vi "VFH Vi.vi"(0 "LIDAR & Vision magn. (m)":dbl[](array[numeric]), 5 "LIDAR & Vision angle (rad)":dbl[](array[numeric]), 7 "current heading (rad)":dbl, 9 "target heading (rad)":dbl, 12 "obstacle clearance (m)":dbl, 13 "thresholds":T1) -> (8 "command heading (rad)":dbl, 10 "histogram out":dbl[](array[numeric]), 15 "mask out":bool[](array[boolean]))   [LabVIEW 2016]
uses:
  <vilib>/Utility/AngleManip/Degrees to Radians (Scalar DBL).vi
  <vilib>/robotics/Obstacle Avoidance/Advanced Vector Field Histogram/NI_Robotics_Vector Field Histogram.lvlib
  <vilib>/Utility/AngleManip/NI_AngleManipulation.lvlib
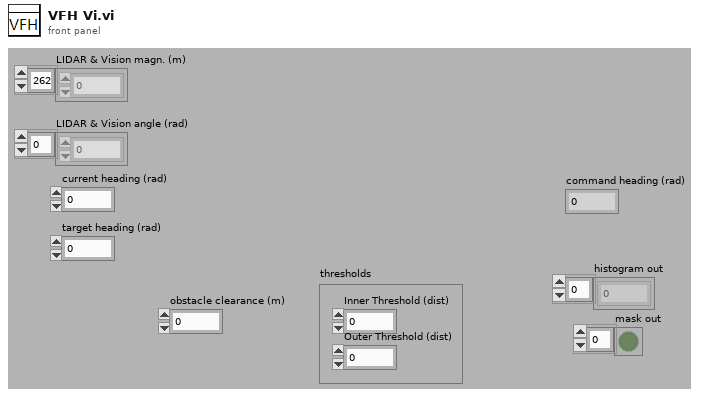
[diagram p1: front panel]
types:
  T1 = cluster{"Inner Threshold (dist)":dbl, "Outer Threshold (dist) ":dbl}
  T2 = cluster{"current heading (rad)":dbl, "target heading (rad)":dbl}
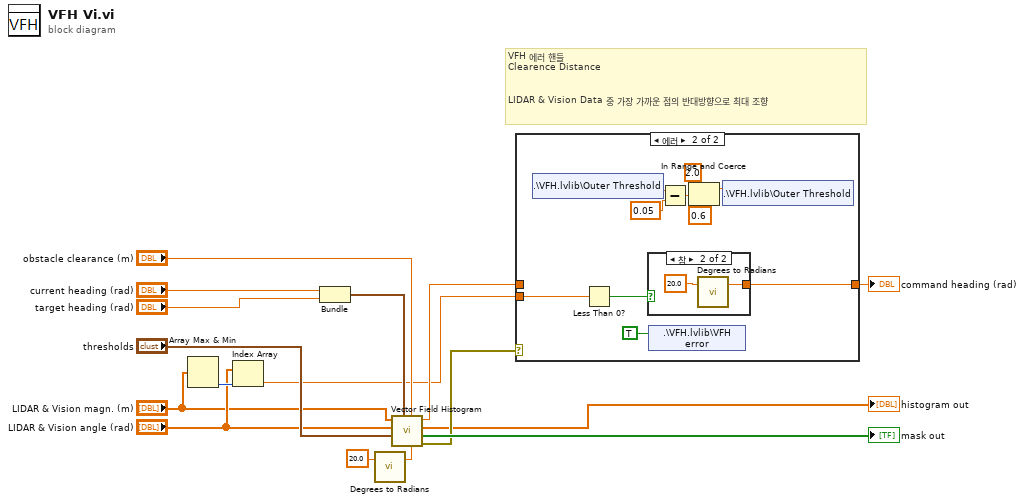
[diagram p0: block diagram]
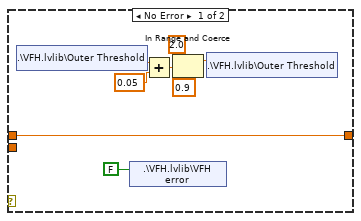
[diagram p2: hidden frame]
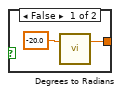
[diagram p3: hidden frame]
diagram:
  # "VFH 에러 핸들\nClearence Distance\n\n\nLIDAR & Vision Data 중 가장 가까운 점의 반대방향으로 최대 조향"
  n1 = Array Max & Min(array="LIDAR & Vision magn. (m)") -> (min index (indices)=w4:i32)  [unwired: 3 out]
  n2 = Index Array(array="LIDAR & Vision angle (rad)", index=w4) -> (element=w2:dbl)
  n3 = Bundle("current heading (rad)"="current heading (rad)", "target heading (rad)"="target heading (rad)") -> (w10:T2)  [unwired: 1 in]
  n4 = call-poly <vilib>:"Degrees to Radians.vi"("angle (deg)"=20.0) -> ("angle (rad)"=w8:dbl)  [unwired: 2 in]
  n5 = call <vilib>:"Vector Field Histogram.vi"("maximum heading change (rad)"=w8, "obstacle clearance distance"="obstacle clearance (m)", "heading"=w10, "thresholds"="thresholds", "direction angles (rad)"="LIDAR & Vision angle (rad)", "distances"="LIDAR & Vision magn. (m)") -> ("error out"=w11:errorcluster, "mask"=→"mask out":bool[], "histogram"=→"histogram out":dbl[], "chosen heading (rad)"=w12:dbl)  [unwired: 2 in]
  n6 = case shown="에러" w11 {
    tunnel: w12 -> [w24 _]
    tunnel: [w24 w32] -> w6
    tunnel: w2 -> [_ w31]
    frame No Error {
      n7 = shared-variable ".\\VFH.lvlib\\Outer Threshold"() -> (w17:dbl)  [unwired: 1 in, 1 out]
      n8 = shared-variable ".\\VFH.lvlib\\VFH error"(FALSE ("VFH error")) -> ()  [unwired: 1 in, 1 out]
      n9 = Add(x=w17, y=0.05) -> (x+y=w21:dbl)
      n10 = In Range and Coerce(upper limit=2.0 ("상위 리미트"), x=w21, lower limit=0.9 ("하위 리미트")) -> (coerced(x)=w22:dbl)  [unwired: 1 out]
      n11 = shared-variable ".\\VFH.lvlib\\Outer Threshold"(w22) -> ()  [unwired: 1 in, 1 out]
    }
    frame Error {
      n12 = shared-variable ".\\VFH.lvlib\\Outer Threshold"() -> (w25:dbl)  [unwired: 1 in, 1 out]
      n13 = Less Than 0?(x=w31) -> (x < 0?=w33:bool)
      n14 = case shown="참" w33 {
        tunnel: [w35 w37] -> w32
        frame False {
          n15 = call-poly <vilib>:"Degrees to Radians.vi"("angle (deg)"=-20.0) -> ("angle (rad)"=w35:dbl)  [unwired: 2 in]
        }
        frame True {
          n16 = call-poly <vilib>:"Degrees to Radians.vi"("angle (deg)"=20.0) -> ("angle (rad)"=w37:dbl)  [unwired: 2 in]
        }
      }
      n17 = shared-variable ".\\VFH.lvlib\\VFH error"(TRUE ("VFH error")) -> ()  [unwired: 1 in, 1 out]
      n18 = Subtract(x=w25, y=0.05) -> (x-y=w29:dbl)
      n19 = In Range and Coerce(upper limit=2.0 ("상위 리미트"), x=w29, lower limit=0.6 ("하위 리미트")) -> (coerced(x)=w30:dbl)  [unwired: 1 out]
      n20 = shared-variable ".\\VFH.lvlib\\Outer Threshold"(w30) -> ()  [unwired: 1 in, 1 out]
    }
  }
  "command heading (rad)" <- w6
